vi "Split recorder block item from answer.vi"(0 "Slice block item":i32 min=1 max=4 step=1, 2 "RecorderIDs to query":string[](array[string]), 4 "Input string":string, 5 "error in":errorcluster) -> (14 "Sliced text segments":string[](array[string]), 19 "error out":errorcluster)   [LabVIEW 2026]
doc: "Slice specific recorder answer into text segments."
panel:
  # "Slice specific recorder answer into text segments."
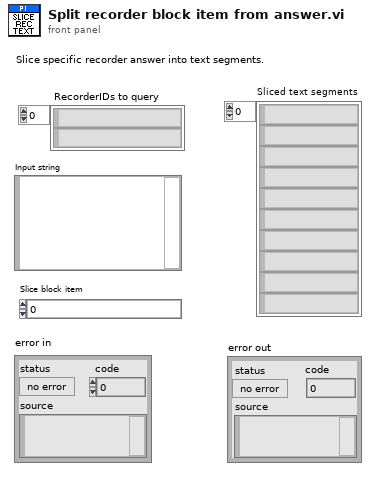
[diagram p1: front panel]
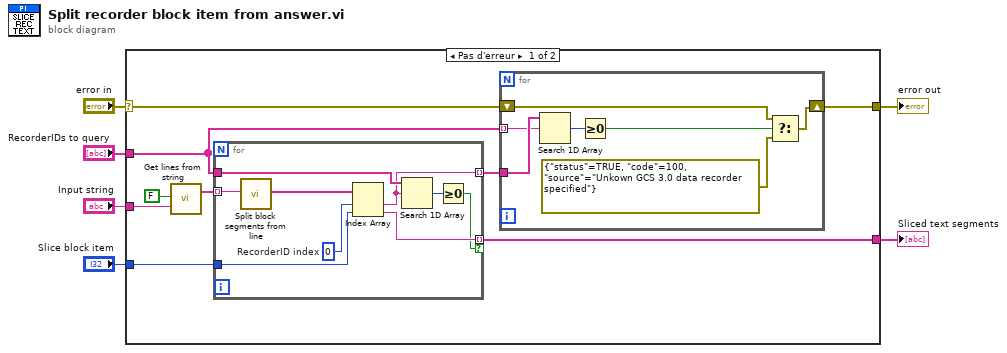
[diagram p0: block diagram]
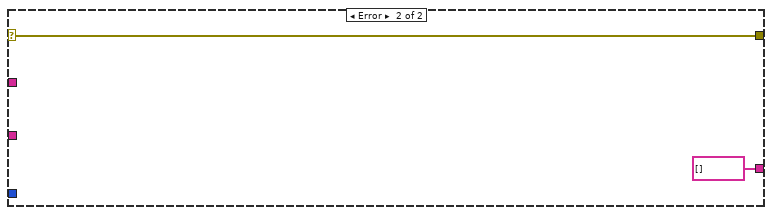
[diagram p2: hidden frame]
diagram:
  n1 = case shown="Pas d'erreur" "error in" {
    selector: "error in" -> [w7 w33]
    tunnel: [w10 w33] -> w5
    tunnel: "RecorderIDs to query" -> [w9 _]
    tunnel: [w13 string[] [] ("Sliced text segments")] -> w3
    tunnel: "Slice block item" -> [w12 _]
    tunnel: "Input string" -> [w11 _]
    frame No Error {
      n2 = call "Get lines from string.vi"("Cut spaces?"=FALSE, "Input string"=w11) -> ("Strings"=w15:string[])  [unwired: 16 in, 1 out]
      n3 = for {
        tunnel: w15 -> [w30] mode=indexing
        tunnel: w12 -> [w29]
        tunnel: [w28] -> w13 mode=indexing if=w25
        tunnel: w9 -> [w26]
        tunnel: [w23] -> w8 mode=indexing
        w27 = 0  # RecorderID index
        n4 = call "Split block segments from line.vi"("Input line string"=w30) -> ("Text segments"=w31:string[])  [unwired: 18 in]
        n5 = Index Array(array=w31, index #1=w27, index #2=w29) -> (element #1=w23:string, element #2=w28:string)
        n6 = Search 1D Array(1D array=w26, element=w23) -> (index of element=w24:i32)  [unwired: 1 in]
        n7 = Greater Or Equal To 0?(x=w24) -> (x >= 0?=w25:bool)
      }
      n8 = for {
        shift-right: [w17] -> w10
        shift-left: w7 -> [w18]
        tunnel: w9 -> [w21] mode=indexing
        tunnel: w8 -> [w22]
        n9 = Search 1D Array(1D array=w22, element=w21) -> (index of element=w20:i32)  [unwired: 1 in]
        n10 = Greater Or Equal To 0?(x=w20) -> (x >= 0?=w19:bool)
        n11 = Select(t=w18, s=w19, f=errorcluster {"status"=TRUE, "code"=100, "source"="Unkown GCS 3.0 data recorder specified"} ("error out")) -> (s? t:f=w17:errorcluster)
      }
    }
    frame Error {
    }
  }
  "error out" <- w5
  "Sliced text segments" <- w3
